vi "Player Info.vi"(11 "AndrewF in":refnum<class "AndrewF.lvclass">) -> (0 "Defeat Speech":string="Don't be a sore winner.", 1 "Victory Speech":string="I win, too bad for you.", 2 "Name":string="Back attack", 3 "AndrewF out":refnum<class "AndrewF.lvclass">)   [LabVIEW 2015, in "AndrewF.lvclass"]
uses:
  AndrewF.lvclass
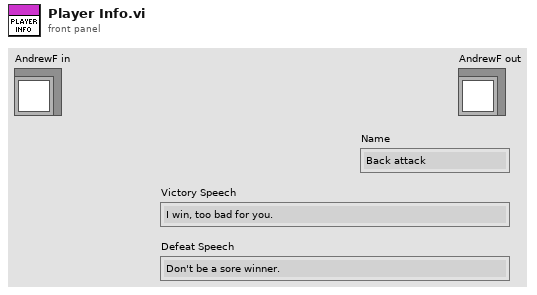
[diagram p1: front panel]
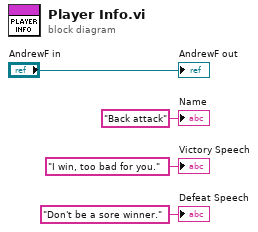
[diagram p0: block diagram]
diagram:
  "AndrewF out" <- "AndrewF in"
  "Name" <- "Back attack" ("Name")
  "Victory Speech" <- "I win, too bad for you." ("Victory Speech")
  "Defeat Speech" <- "Don't be a sore winner." ("Defeat Speech")
